vi "Pendel mit statechart.vi"() -> ()   [LabVIEW 2013]
uses:
  Pendel.lvsc/Trigger.ctl
  Pendel.lvsc
  <vilib>/Statechart/Nodes/EventFiring/NI_SC_EventFiringNode.xnode
  <vilib>/Statechart/Infrastructure/RTStatechart/RunTime SCN.xnode
  Pendel.lvsc/Outputs.ctl
  Pendel.lvsc/Inputs.ctl
  <vilib>/CANopenLib/CANOPEN.llb/CANopen BaudRate.ctl
panel:
  in  "Registerkarte":enum32{"Haupt", "Einstellungen"}(tab)
  out "Winkelgeschwindigkeit1":dbl
  out "Winkel 1":dbl
  out "Geschwindigkeit":dbl
  out "Position":dbl
  in  "Schließen":bool
  in  "Stop Regler":bool
  in  "Start Regler":bool
  in  "Ruhelage":bool
  in  "Pendelaufbau":enum16{"Einfachpendel", "Doppelpendel"}(ring)
  in  "Regler":enum16{""}(ring)
  out "Aktueller Zustand":string
  in  "Referenzieren":bool
  in  "Einstellungen":T2={"CANopen-Optionen"={"CANopen Interface"=0, "node-ID"=2, "Baud Rate"=0}} {"CANopen-Optionen"."Baud Rate" items=["1 Mbit/s"=0, "800 kbit/s"=1, "500 kbit/s"=2, "250 kbit/s"=3, "125 kbit/s"=4, "50 kbit/s"=6, "20 kbit/s"=7, "10 kbit/s"=8]; "CANopen-Optionen"."CANopen Interface" items=["CANopen01", "CANopen02", "CANopen03", "CANopen04", "CANopen05", "CANopen06", "CANopen07", "CANopen08", "CANopen09", "CANopen10", "CANopen11", "CANopen12", "CANopen13", "CANopen14", "CANopen15", "CANopen16", "CANopen17", "CANopen18", "CANopen19", "CANopen20", "CANopen21", "CANopen22", "CANopen23", "CANopen24", "CANopen25", "CANopen26", "CANopen27", "CANopen28", "CANopen29", "CANopen30", "CANopen31", "CANopen32"]}
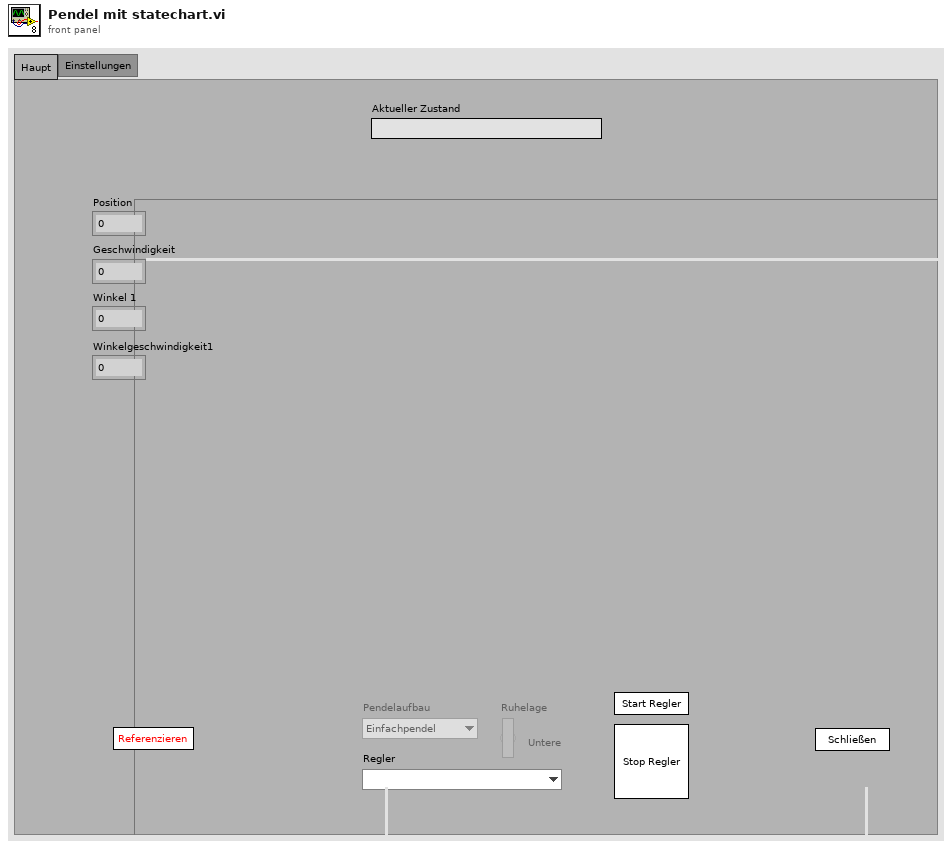
[diagram p1: front panel]
types:
  T1 = typedef "CANopen BaudRate.ctl" = u32
  T2 = cluster{"CANopen-Optionen":cluster{"CANopen Interface":u32, "node-ID":u8, "Baud Rate":T1}}
  T3 = cluster{"Einstellungen":cluster{"CANopen-Optionen":cluster{"CANopen Interface":u32, "node-ID":u8, "Baud Rate":T1}}, "Regler":enum16{""}}
  T4 = typedef "Pendel.lvsc/Inputs.ctl" = cluster{"Referenzieren":bool, "Regler starten":bool, "Regler anhalten":bool, "Schließen":bool, "error in (no error)":errorcluster}
  T5 = typedef "Pendel.lvsc/Outputs.ctl" = cluster{"Zustand":string, "Regler aktiv":bool, "error out":errorcluster}
  T6 = typedef "Pendel.lvsc/Trigger.ctl" = enum16{"NULL"}
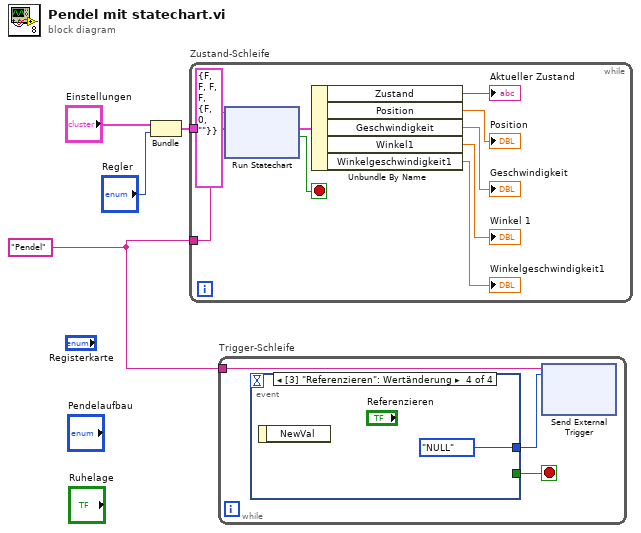
[diagram p0: block diagram]
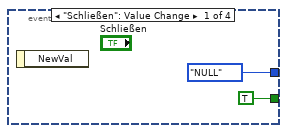
[diagram p2: hidden frame]
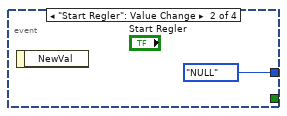
[diagram p3: hidden frame]
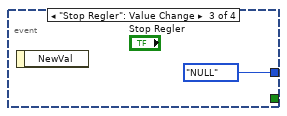
[diagram p4: hidden frame]
diagram:
  w1 = "Pendel" ("Instance Name")
  n1 = Bundle("Einstellungen"="Einstellungen", "Regler"="Regler") -> (w3:T3)  [unwired: 1 in]
  n2 = while "Zustand-Schleife" {
    tunnel: w3 -> [_]
    tunnel: w1 -> [w6]
    stop <- w7 stop-if-true
    n3 = xnode "Run Statechart"("Inputs"=T4 {"Referenzieren"=FALSE, "Regler starten"=FALSE, "Regler anhalten"=FALSE, "Schließen"=FALSE, "error in (no error)"={"status"=FALSE, "code"=0, "source"=""}}, "Trigger"=w6) -> ("Terminated?"=w7:bool, "Outputs"=w13:T5)  [unwired: 1 in]
    n4 = Unbundle By Name(w13) -> ("Zustand"=→"Aktueller Zustand":string, "Position"=→"Position":dbl, "Geschwindigkeit"=→"Geschwindigkeit":dbl, "Winkel1"=→"Winkel 1":dbl, "Winkelgeschwindigkeit1"=→"Winkelgeschwindigkeit1":dbl)
  }
  n5 = while "Trigger-Schleife" {
    tunnel: w1 -> [w15]
    stop <- w14 stop-if-true
    n6 = event shown="[3] \"Referenzieren\": Wertänderung" {
      selector: _ -> [_ _ _ _]
      dyn-events: _ -> [_ _ _ _]
      timeout: _ -> [_ _ _ _]
      tunnel: [Trigger."NULL" ("Trigger") Trigger."NULL" ("Trigger") Trigger."NULL" ("Trigger") Trigger."NULL" ("Trigger")] -> w16
      tunnel: [TRUE _ _ _] -> w14
      event "Schließen": Value Change {
        n7 = event-data() -> ()  [unwired: 1 in, 1 out]
      }
      event "Start Regler": Value Change {
        n8 = event-data() -> ()  [unwired: 1 in, 1 out]
      }
      event "Stop Regler": Value Change {
        n9 = event-data() -> ()  [unwired: 1 in, 1 out]
      }
      event "Referenzieren": Value Change {
        n10 = event-data() -> ()  [unwired: 1 in, 1 out]
      }
    }
    n11 = xnode "Send External Trigger"("Instance Name"=w15, "Trigger"=w16) -> ()  [unwired: 1 in, 2 out]
  }
